vi "AlliGator Get Phasor Plot Data.vi"(8 "error in (no error)":errorcluster, 10 "Plot Idx (-1: last)":i32=-1, 11 "Phasor Graph Refnum":refnum<vi>) -> (0 "error out":errorcluster, 1 "Plot Name":string, 2 "Plot Idx":i32, 3 "Phasor Array":T1[](array[typedef]))   [LabVIEW 2021, in "AlliGator Phasor Graph.lvlib"]
doc: "Returns the phasors in the selected phasor plot."
uses:
  AlliGator Phasor Graph.lvlib
  Phasor/Phasor (g, s).ctl
  Phasor/Phasor.lvlib
  Arrays/Arrays.lvlib
  Graphs/XY Graph/XY Graph Add-Ons.lvlib
panel:
  # "see the AlliGator License on the block diagram (Ctrl+E or Window:Show Block Diagram)"
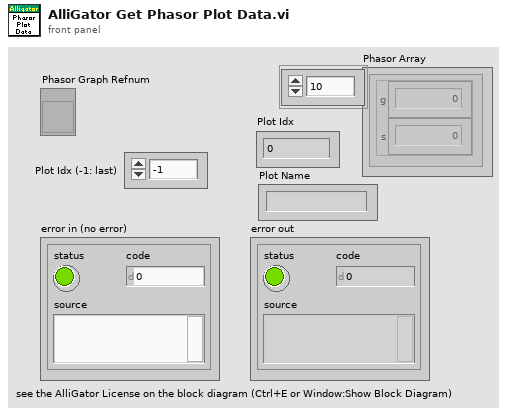
[diagram p1: front panel]
types:
  T1 = typedef "Phasor.lvlib/Phasor (g, s).ctl" = cluster{"g":dbl, "s":dbl}
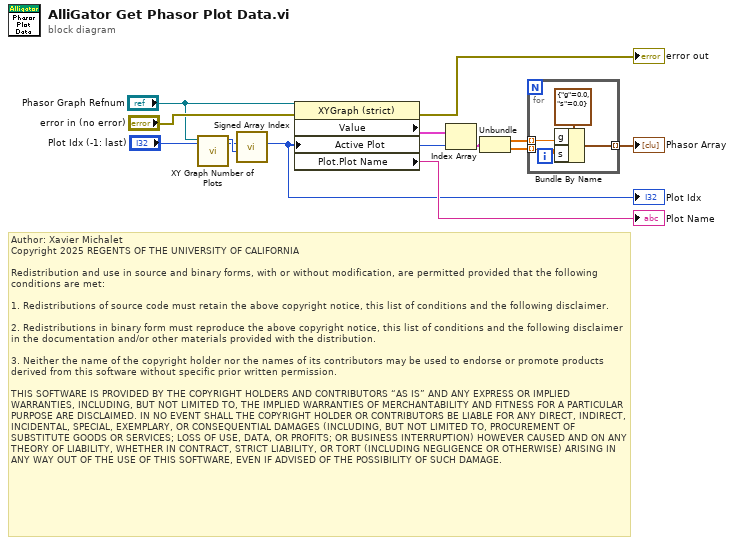
[diagram p0: block diagram]
diagram:
  # "Author: Xavier Michalet\nCopyright 2025 REGENTS OF THE UNIVERSITY OF CALIFORNIA\n\nRedistribution and use in source and binary forms, with or without modification, are permitted provided that the following conditions are met:\n\n1. Redistributions of source code must retain the above copyright notice, this list of conditions and the following disclaimer.\n\n2. Redistributions in binary form must reproduce the above copyright notice, this list of conditions and the following disclaimer in the documentation and/or other materials provided with the distribution.\n\n3. Neither the name of the copyright holder nor the names of its contributors may be used to endorse or promote products derived from this software without specific prior written permission.\n\nTHIS SOFTWARE IS PROVIDED BY THE COPYRIGHT HOLDERS AND CONTRIBUTORS “AS IS” AND ANY EXPRESS OR IMPLIED WARRANTIES, INCLUDING, BUT NOT LIMITED TO, THE IMPLIED WARRANTIES OF MERCHANTABILITY AND FITNESS FOR A PARTICULAR PURPOSE ARE DISCLAIMED. IN NO EVENT SHALL THE COPYRIGHT HOLDER OR CONTRIBUTORS BE LIABLE FOR ANY DIRECT, INDIRECT, INCIDENTAL, SPECIAL, EXEMPLARY, OR CONSEQUENTIAL DAMAGES (INCLUDING, BUT NOT LIMITED TO, PROCUREMENT OF SUBSTITUTE GOODS OR SERVICES; LOSS OF USE, DATA, OR PROFITS; OR BUSINESS INTERRUPTION) HOWEVER CAUSED AND ON ANY THEORY OF LIABILITY, WHETHER IN CONTRACT, STRICT LIABILITY, OR TORT (INCLUDING NEGLIGENCE OR OTHERWISE) ARISING IN ANY WAY OUT OF THE USE OF THIS SOFTWARE, EVEN IF ADVISED OF THE POSSIBILITY OF SUCH DAMAGE."
  n1 = call "XY Graph Number of Plots.vi"("XYGraph in"="Phasor Graph Refnum") -> ("# Plots"=w3:i32)  [unwired: 9 in, 1 out]
  n2 = call "Signed Array Index.vi"("Array Size"=w3, "Array Index in"="Plot Idx (-1: last)") -> ("Array Index out"=w1:i32)  [unwired: 9 in]
  "Plot Idx" <- w1
  n3 = property class="XYGraph (strict)"(reference="Phasor Graph Refnum", error in="error in (no error)", "Active Plot"=w1) -> (error out=→"error out":errorcluster, "Value"=w12:cluster{dbl[], dbl[]}[], "Plot.Plot Name"=→"Plot Name":string)  [unwired: 1 out]
  n4 = Index Array(array=w12, index=w1) -> (element=w10:cluster{dbl[], dbl[]})
  n5 = Unbundle(w10) -> (w9:dbl[], w8:dbl[])
  n6 = for {
    tunnel: w9 -> [w13] mode=indexing
    tunnel: w8 -> [w14] mode=indexing
    tunnel: [w15] -> w7 mode=indexing
    n7 = Bundle By Name(cluster=T1 {"g"=0.0, "s"=0.0} ("Phasor"), "g"=w13, "s"=w14) -> (w15:T1)
  }
  "Phasor Array" <- w7
